vi "InterpretBD.vi"(6 "error in":errorcluster, 9 "VI Interpreter in":refnum<class "VI Interpreter.lvclass">) -> (0 "error out":errorcluster, 3 "VI Interpreter out":refnum<class "VI Interpreter.lvclass">)   [LabVIEW 2014, in "VI Interpreter.lvclass"]
uses:
  VI Interpreter.lvclass
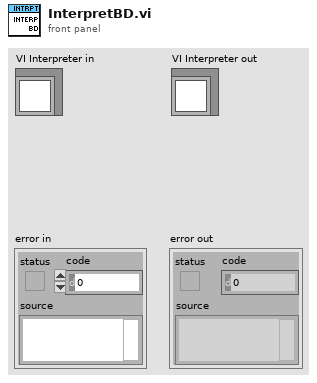
[diagram p1: front panel]
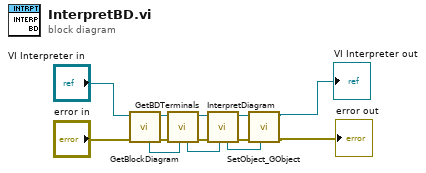
[diagram p0: block diagram]
diagram:
  n1 = call "GetBlockDiagram.vi"("error in"="error in", "VI Interpreter in"="VI Interpreter in") -> ("error out"=w12:errorcluster, "VI Interpreter out"=w13:refnum<class "VI Interpreter.lvclass">, "TopLevelDiagram"=w11:refnum<class "TopLevelDiagram.lvclass">)  [unwired: 5 in]
  n2 = call "GetBDTerminals.vi"("Diagram"=w11, "error in"=w12, "VI Interpreter in"=w13) -> ("error out"=w9:errorcluster, "VI Interpreter out"=w10:refnum<class "VI Interpreter.lvclass">, "Diagram out"=w8:refnum<class "TopLevelDiagram.lvclass">)  [unwired: 4 in]
  n3 = call "InterpretDiagram.vi"("Diagram"=w8, "error in"=w9, "VI Interpreter in"=w10) -> ("error out"=w6:errorcluster, "VI Interpreter out"=w7:refnum<class "VI Interpreter.lvclass">, "Diagram out"=w1:refnum<class "TopLevelDiagram.lvclass">)  [unwired: 4 in]
  n4 = call "SetObject_GObject.vi"("GObject"=w1, "error in"=w6, "VI Interpreter in"=w7) -> ("error out"=→"error out":errorcluster, "VI Interpreter out"=→"VI Interpreter out":refnum<class "VI Interpreter.lvclass">)  [unwired: 5 in]
